vi "Register Groups.vi"(8 "error in (no error)":errorcluster, 9 "Promise":refnum<class "Promise.lvclass">, 10 "Groups":refnum<class "Group.lvclass">[](array[class]), 11 "DataHandlerTask in":refnum<class "DataHandlerTask.lvclass">) -> (0 "error out":errorcluster, 3 "DataHandlerTask out":refnum<class "DataHandlerTask.lvclass">)   [LabVIEW 2020, in "VolatusData.lvlib" / "DataHandlerTask.lvclass"]
uses:
  DataHandlerTask.lvclass
  lv-vecto/Vecto/GroupAbstract/GroupAbstract.lvclass
  lv-promises/Promises/Promise/Promise.lvclass
  lv-promises/Promises/Error Result/Error Result.lvclass
  Volatus/Task/Task.lvclass
  lv-vecto/Vecto/Group/Group.lvclass
  C:/dev/lv20CE/relink/lv-vecto/Vecto/GroupAbstract/GroupAbstract.lvclass
  C:/dev/lv20CE/relink/lv-vecto/Vecto/Group/Group.lvclass
  C:/dev/lv20CE/relink/lv-promises/Promises/Value/Value.lvclass
  C:/dev/lv20CE/relink/lv-promises/Promises/Error Result/Error Result.lvclass
  C:/dev/lv20CE/relink/lv-volatus/Volatus/Task/Task.lvclass
  C:/Program Files (x86)/National Instruments/LabVIEW 2020/vi.lib/ActorFramework/Actor/Actor.lvclass
  C:/dev/lv20CE/relink/lv-volatus/Volatus/TaskStateHandler/TaskStateHandler.lvclass
  C:/dev/lv20CE/relink/lv-volatus/Volatus/VectoMessageHandler/VectoMessageHandler.lvclass
  C:/dev/lv20CE/relink/lv-volatus/Volatus/DataHandlerTask/DataHandlerTask.lvclass
  C:/dev/lv20CE/relink/lv-volatus/Volatus/API Provider/API Provider.lvclass
  C:/dev/lv20CE/relink/lv-volatus/Volatus/DataHandler/DataHandler.lvclass
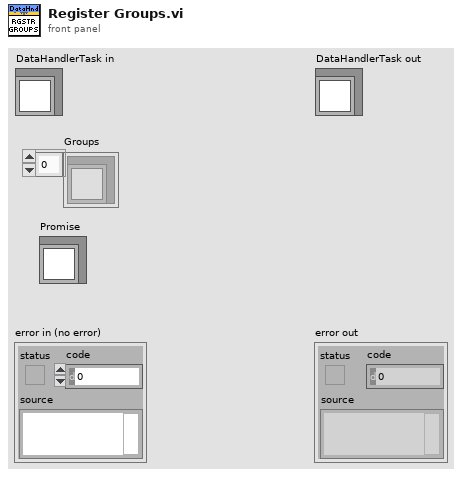
[diagram p1: front panel]
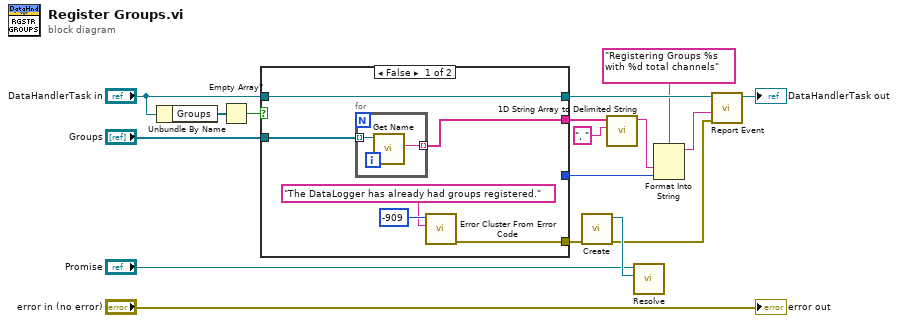
[diagram p0: block diagram]
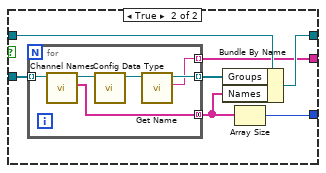
[diagram p2: hidden frame]
diagram:
  n1 = Unbundle By Name("DataHandlerTask in") -> ("Groups"=w16:refnum<class "Group.lvclass">[])
  n2 = Empty Array?(array=w16) -> (empty?=w13:bool)
  n3 = case shown="False" w13 {
    tunnel: "Groups" -> [w19 w32]
    tunnel: [w23 w31] -> w11
    tunnel: "DataHandlerTask in" -> [w23 w29]
    tunnel: [w20 _] -> w15
    tunnel: [w18 w28] -> w7
    tunnel: [_ w26] -> w2
    frame False {
      n4 = for {
        tunnel: w19 -> [w25] mode=indexing
        tunnel: [w24] -> w18 mode=indexing
        n5 = call "Get Name.vi"("GroupAbstract in"=w25) -> ("Name"=w24:string)  [unwired: 8 in, 2 out]
      }
      n6 = call <vilib>:"Error Cluster From Error Code.vi"("error message (\"\")"="The DataLogger has already had groups registered.", "error code (0)"=-909) -> ("error out"=w20:errorcluster)  [unwired: 7 in]
    }
    frame True {
      n7 = for {
        tunnel: w32 -> [w33] mode=indexing
        tunnel: [w35] -> w30 mode=indexing
        tunnel: [w37] -> w27 mode=concatenating
        tunnel: [w34] -> w28 mode=indexing
        n8 = call "Channel Names.vi"("GroupAbstract in"=w33) -> ("Channel Names"=w37:string[], "GroupAbstract out"=w38:refnum<class "Group.lvclass">)  [unwired: 8 in, 1 out]
        n9 = call "Config Data Type.vi"("GroupAbstract in"=w38) -> ("GroupAbstract out"=w36:refnum<class "Group.lvclass">)  [unwired: 8 in, 2 out]
        n10 = call "Get Name.vi"("GroupAbstract in"=w36) -> ("Name"=w34:string, "GroupAbstract out"=w35:refnum<class "Group.lvclass">)  [unwired: 8 in, 1 out]
      }
      n11 = Bundle By Name(cluster=w29, "Groups"=w30, "Names"=w27) -> (w31:refnum<class "DataHandlerTask.lvclass">)
      n12 = Array Size(array=w27) -> (size(s)=w26:i32)
    }
  }
  n13 = call "Create.vi"("error in (no error)"=w15) -> ("error out"=w5:errorcluster, "Error Result out"=w14:refnum<class "Error Result.lvclass">)  [unwired: 9 in]
  n14 = call <vilib>:"1D String Array to Delimited String.vi"("delimiter"=", ", "string array"=w7) -> ("delimited string"=w3:string)  [unwired: 9 in]
  n15 = call "Resolve.vi"("Result"=w14, "Promise in"="Promise") -> ()  [unwired: 8 in, 2 out]
  n16 = Format Into String(format string="Registering Groups %s with %d total channels", w3, w2) -> (resulting string=w1:string)  [unwired: 2 in, 1 out]
  n17 = call "Report Event.vi"("error in (no error)"=w5, "Message"=w1, "Task in"=w11) -> ("Task in"=→"DataHandlerTask out":refnum<class "DataHandlerTask.lvclass">)  [unwired: 7 in, 1 out]
  "error out" <- "error in (no error)"
